vi "Write Prefix.vi"(8 "error in (no error)":errorcluster, 10 "Prefix":string, 11 "Lakeshore 325 in":refnum<class "Lakeshore 325.lvclass">) -> (0 "error out":errorcluster, 3 "Lakeshore 325 out":refnum<class "Lakeshore 325.lvclass">)   [LabVIEW 2022 SP3, in "Lakeshore 325.lvclass"]
uses:
  Lakeshore 325.lvclass
  Lakeshore 325.lvclass/Lakeshore 325.ctl
  Temp Control.lvclass
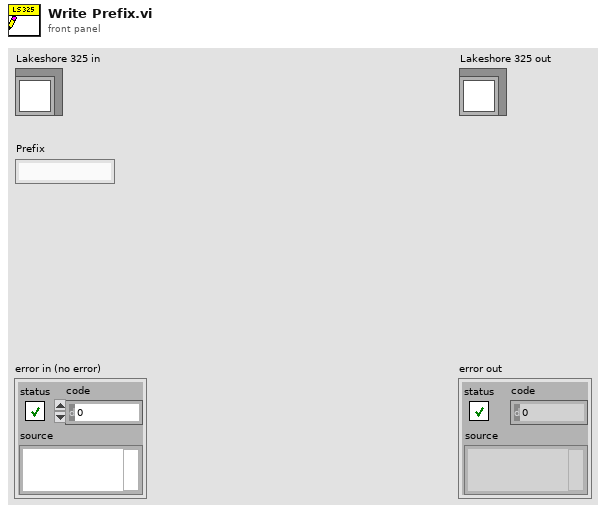
[diagram p1: front panel]
types:
  T1 = typedef "Lakeshore 325.lvclass/Lakeshore 325 Settings cluster.ctl" = cluster{"Addr":refnum<visa-resource-name>, "Ch Prefix":string, "Ch Select":i32[]}
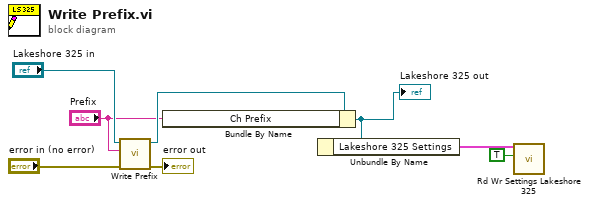
[diagram p0: block diagram]
diagram:
  n1 = call-parent "Write Prefix.vi"("error in (no error)"="error in (no error)", "Prefix"="Prefix", "Temp Control in"="Lakeshore 325 in") -> ("error out"=→"error out":errorcluster, "Temp Control out"=w5:refnum<class "Lakeshore 325.lvclass">)  [unwired: 7 in]
  n2 = Bundle By Name(cluster=w5, "Ch Prefix"="Prefix") -> (w3:refnum<class "Lakeshore 325.lvclass">)
  "Lakeshore 325 out" <- w3
  n3 = Unbundle By Name(w3) -> ("Lakeshore 325 Settings"=w2:T1)
  n4 = call "Rd Wr Settings Lakeshore 325.vi"("Write? (F:Read)"=TRUE, "Lakeshore 325 Settings"=w2) -> ()  [unwired: 8 in, 2 out]
